vi "one-hot.vi"(1 "array":dbl[](array[numeric])) -> (0 "transposed array":dbl[][](array[numeric]))   [LabVIEW 2023]
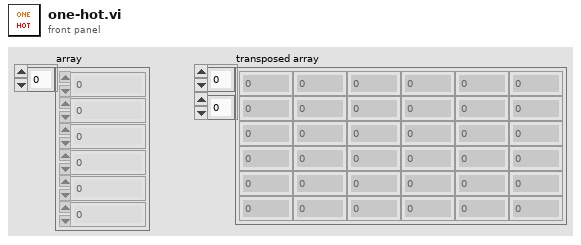
[diagram p1: front panel]
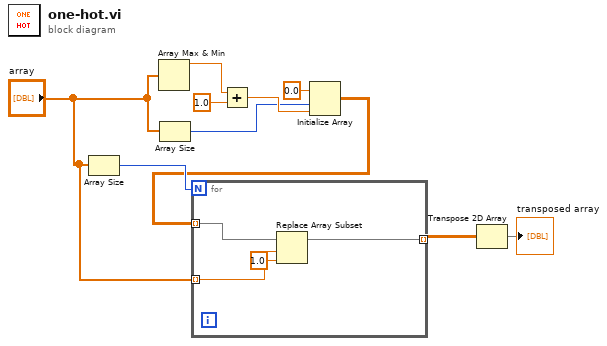
[diagram p0: block diagram]
diagram:
  n1 = Array Size(array="array") -> (size(s)=w7:i32)
  n2 = Array Max & Min(array="array") -> (max value=w3:dbl)  [unwired: 3 out]
  n3 = Array Size(array="array") -> (size(s)=w1:i32)
  n4 = Add(x=w3, y=1.0) -> (x+y=w4:dbl)
  n5 = Initialize Array(0.0 ("element"), w1, w4) -> (w6:dbl[][])
  n6 = for {
    N: w7 -> [_]
    tunnel: w6 -> [w14] mode=indexing
    tunnel: "array" -> [w13] mode=indexing
    tunnel: [w11] -> w9 mode=indexing
    n7 = Replace Array Subset(array=w14, new element=1.0 ("new element/subarray"), index=w13) -> (w11:dbl[])
  }
  n8 = Transpose 2D Array(2D array=w9) -> (transposed array=→"transposed array":dbl[][])
